vi "wave.vi"() -> ()   [LabVIEW 2020]
uses:
  <vilib>/measure/NI_MABase.lvlib
panel:
  out "Waveform Graph":waveform(dbl)(graph)
  in  "Frequency":dbl(knob) scale=0.0..100.0
  in  "Amplitude":dbl(knob) scale=0.0..10.0
  in  "Signal Type":enum16{"Square", "Sine", "Saw", "Triangular"}(ring)
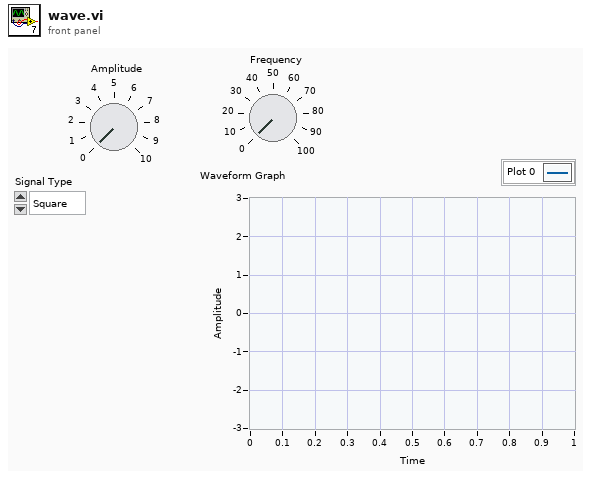
[diagram p1: front panel]
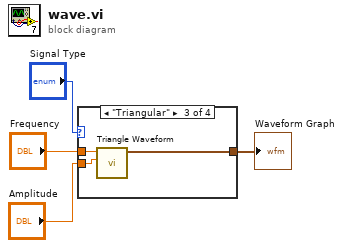
[diagram p0: block diagram]
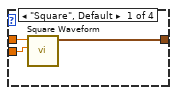
[diagram p2: hidden frame]
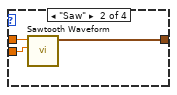
[diagram p3: hidden frame]
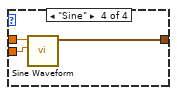
[diagram p4: hidden frame]
diagram:
  n1 = case shown="\"Triangular\"" "Signal Type" {
    tunnel: "Frequency" -> [w7 w9 w12 w16]
    tunnel: "Amplitude" -> [w6 w8 w11 w15]
    tunnel: [w5 w10 w13 w14] -> w1
    frame "Square", Default {
      n2 = call <vilib>:"Square Waveform.vi"("amplitude"=w6, "frequency"=w7) -> ("signal out"=w5:waveform(dbl))  [unwired: 8 in, 1 out]
    }
    frame "Saw" {
      n3 = call <vilib>:"Sawtooth Waveform.vi"("amplitude"=w8, "frequency"=w9) -> ("signal out"=w10:waveform(dbl))  [unwired: 8 in, 1 out]
    }
    frame "Triangular" {
      n4 = call <vilib>:"Triangle Waveform.vi"("amplitude"=w11, "frequency"=w12) -> ("signal out"=w13:waveform(dbl))  [unwired: 8 in, 1 out]
    }
    frame "Sine" {
      n5 = call <vilib>:"Sine Waveform.vi"("amplitude"=w15, "frequency"=w16) -> ("signal out"=w14:waveform(dbl))  [unwired: 8 in, 1 out]
    }
  }
  "Waveform Graph" <- w1
